vi "Xml_Save_Sequence.vi"(8 "error in (no error)":errorcluster, 11 "Refnum Clust":refnum<vi>) -> (0 "error out":errorcluster, 3 "XML String Out":string[](array[string]))   [LabVIEW 2018]
uses:
  controls/SEQUENCE_Inputs.ctl
  controls/EXCIT_Inputs.ctl
  controls/DATA_Inputs.ctl
  controls/TIMING_Inputs.ctl
  controls/PROCESSING_Inputs.ctl
  controls/TRAPPING_Inputs.ctl
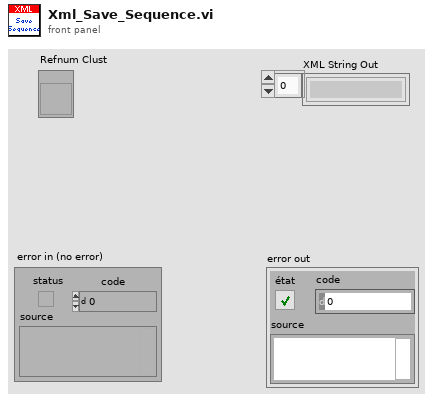
[diagram p1: front panel]
types:
  T1 = typedef "SEQUENCE_Inputs.ctl" = cluster{"EXCIT Inputs":T2, "DATA Inputs":T3, "TIMING Inputs":T4, "PROCESSING Inputs":T5, "TRAPPING Inputs":T6}
  T2 = typedef "EXCIT_Inputs.ctl" = cluster{"Number of Excitations":i32, "Script Text":string, "Table of Waveforms":string[]}
  T3 = typedef "DATA_Inputs.ctl" = cluster{"Record Length":i32, "Sample Rate":dbl, "Data Type":u8, "Vertical Range":dbl, "Acquisition Duration":dbl}
  T4 = typedef "TIMING_Inputs.ctl" = cluster{"Number of Acquisitions ":i16, "Number of Accumulations":i16, "Table of Waveforms":string[], "Script Text":string}
  T5 = typedef "PROCESSING_Inputs.ctl" = cluster{"Reference Mass":dbl, "Cyclotron Freq":dbl, "Magnetron Freq":dbl}
  T6 = typedef "TRAPPING_Inputs.ctl" = cluster{"Number of Channels":i32, "Init Values":dbl[], "Opening Values":dbl[], "Trapping Values":dbl[], "Emptying Values":dbl[], "Adiabatic ON":bool, "Adiabatic Duration":i32, "Adiabatic Waveforms":string[], "Ions Refill ON":bool, "Number of Ions Refills":i32, "Trapping Delay":dbl, "Trapping Duration":dbl}
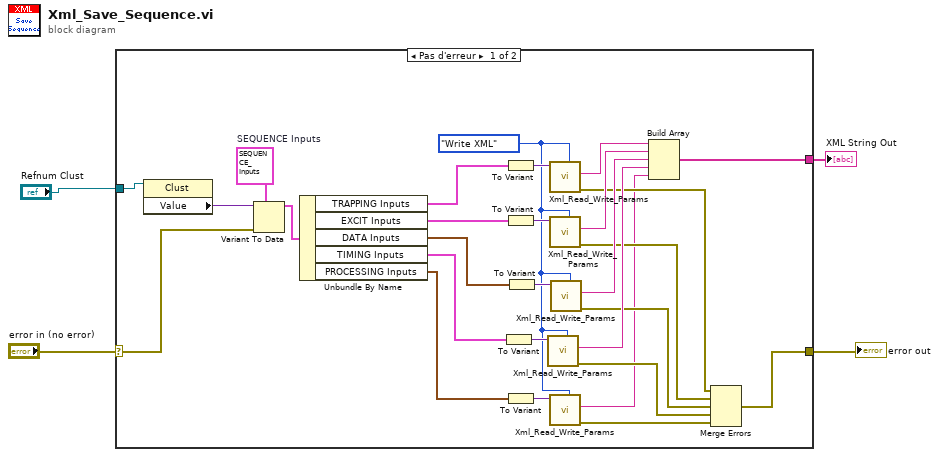
[diagram p0: block diagram]
diagram:
  n1 = case shown="Pas d'erreur" "error in (no error)" {
    selector: "error in (no error)" -> [w32 w33]
    tunnel: [w30 w33] -> w3
    tunnel: [w31 _] -> w2
    tunnel: "Refnum Clust" -> [w11 _]
    frame No Error {
      w28 = T1 {"EXCIT Inputs"={"Number of Excitations"=1, "Script Text"="", "Table of Waveforms"=[]}, "DATA Inputs"={"Record Length"=8192, "Sample Rate"=4.0, "Data Type"=0, "Vertical Range"=0.0, "Acquisition Duration"=100000.0}, "TIMING Inputs"={"Number of Acquisitions "=1, "Number of Accumulations"=1, "Table of Waveforms"=[], "Script Text"=""}, "PROCESSING Inputs"={"Reference Mass"=300.0939, "Cyclotron Freq"=255.727, "Magnetron Freq"=0.001}, "TRAPPING Inputs"={"Number of Channels"=4, "Init Values"=[2.0, 5.0, 5.0, 2.0], "Opening Values"=[0.0, 0.0, 0.0, 0.0], "Trapping Values"=[2.0, 5.0, 5.0, 2.0], "Emptying Values"=[-5.0, -5.0, -5.0, -5.0], "Adiabatic ON"=FALSE, "Adiabatic Duration"=0, "Adiabatic Waveforms"=["Adiabatic_None_2_2_2000.bin", "Adiabatic_Ramp_5_0_2000.bin", "Adiabatic_DoubleRamp_5_0_2000.bin", "Adiabatic_RC_2_0_2000.bin"], "Ions Refill ON"=FALSE, "Number of Ions Refills"=4, "Trapping Delay"=400.0, "Trapping Duration"=300.0}}  # SEQUENCE Inputs
      w8 = enum16{"Read XML", "Set", "Get", "Write XML"}."Write XML" ("Command")
      n2 = property class="Clust"(reference=w11) -> ("Value"=w10:variant)  [unwired: 1 in, 2 out]
      n3 = Variant To Data(error in=w32, type=w28, Variant=w10) -> (data=w27:T1)  [unwired: 1 out]
      n4 = Unbundle By Name(w27) -> ("TRAPPING Inputs"=w26:T6, "EXCIT Inputs"=w18:T2, "DATA Inputs"=w17:T3, "TIMING Inputs"=w16:T4, "PROCESSING Inputs"=w7:T5)
      n5 = To Variant(anything=w16) -> (Variant=w23:variant)
      n6 = To Variant(anything=w26) -> (Variant=w29:variant)
      n7 = To Variant(anything=w18) -> (Variant=w25:variant)
      n8 = To Variant(anything=w7) -> (Variant=w9:variant)
      n9 = To Variant(anything=w17) -> (Variant=w24:variant)
      n10 = call "Xml_Read_Write_Params.vi"("Variant"=w23, "Command"=w8) -> ("XML String Out"=w22:string, "error out"=w15:errorcluster)  [unwired: 5 in, 1 out]
      n11 = call "Xml_Read_Write_Params.vi"("Variant"=w29, "Command"=w8) -> ("XML String Out"=w19:string, "error out"=w12:errorcluster)  [unwired: 5 in, 1 out]
      n12 = call "Xml_Read_Write_Params.vi"("Variant"=w25, "Command"=w8) -> ("XML String Out"=w20:string, "error out"=w13:errorcluster)  [unwired: 5 in, 1 out]
      n13 = call "Xml_Read_Write_Params.vi"("Variant"=w9, "Command"=w8) -> ("XML String Out"=w5:string, "error out"=w6:errorcluster)  [unwired: 5 in, 1 out]
      n14 = call "Xml_Read_Write_Params.vi"("Variant"=w24, "Command"=w8) -> ("XML String Out"=w21:string, "error out"=w14:errorcluster)  [unwired: 5 in, 1 out]
      n15 = Build Array(w19, w20, w21, w22, w5) -> (w31:string[])
      n16 = Merge Errors(w12, w13, w14, w15, w6) -> (w30:errorcluster)
    }
    frame Error {
    }
  }
  "error out" <- w3
  "XML String Out" <- w2
